vi "read.vi"(8 "error in (no error)":errorcluster, 11 "Lakeshore 336 in":refnum<class "Lakeshore 336.lvclass">) -> (0 "error out":errorcluster, 2 "Data":dbl[](array[numeric]), 3 "Lakeshore 336 out":refnum<class "Lakeshore 336.lvclass">)   [LabVIEW 2022 SP3, in "Lakeshore 336.lvclass"]
uses:
  Lakeshore 336.lvclass
  Lakeshore 336.lvclass/Lakeshore 336.ctl
  Temp Control.lvclass
  <instrlib>/Lake Shore 336/Lake Shore 336.lvlib
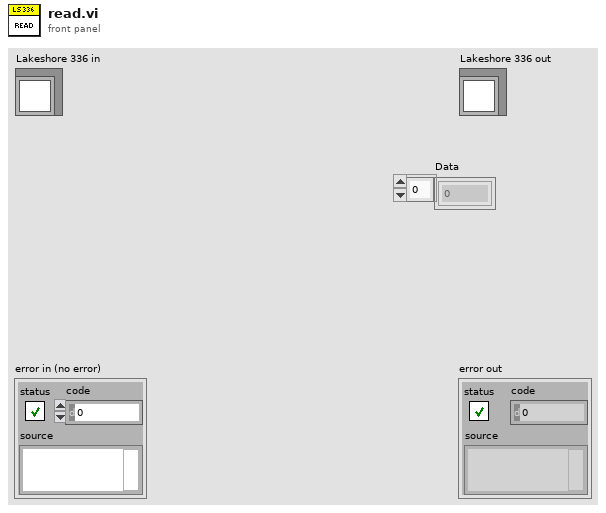
[diagram p1: front panel]
types:
  T1 = typedef "Lakeshore 336.lvclass/Lakeshore 336 Input Ch config cluster.ctl" = cluster{"Name":string}
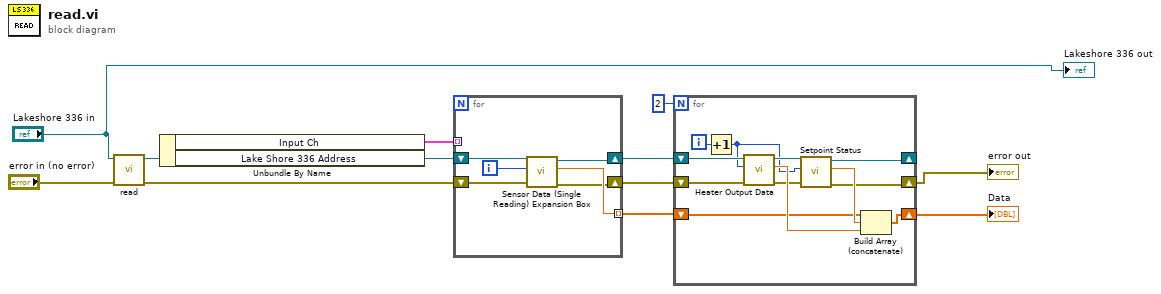
[diagram p0: block diagram]
diagram:
  n1 = call-parent "read.vi"("error in (no error)"="error in (no error)", "Temp Control in"="Lakeshore 336 in") -> ("error out"=w4:errorcluster, "Temp Control out"=w11:refnum<class "Lakeshore 336.lvclass">)  [unwired: 7 in, 1 out]
  n2 = Unbundle By Name(w11) -> ("Input Ch"=w9:T1[], "Lake Shore 336 Address"=w10:refnum<visa-resource-name>)
  n3 = for {
    tunnel: w9 -> [_] mode=indexing
    shift-right: [w16] -> w8
    shift-left: w10 -> [w18]
    tunnel: [w15] -> w6 mode=indexing
    shift-right: [w13] -> w3
    shift-left: w4 -> [w14]
    i -> [w17]
    n4 = call "Sensor Data (Single Reading) Expansion Box.vi"("error in (no error)"=w14, "Input (0:A)"=w17, "VISA resource name"=w18) -> ("error out"=w13:errorcluster, "Sensor Data"=w15:dbl, "VISA resource name out"=w16:refnum<visa-resource-name>)  [unwired: 6 in]
  }
  n5 = for {
    N: 2 -> [_]
    shift-right: [w27] -> _
    shift-left: w8 -> [w30]
    shift-right: [w23] -> w5
    shift-left: w6 -> [w24]
    shift-right: [w20] -> w2
    shift-left: w3 -> [w22]
    i -> [w29]
    n6 = Increment(x=w29) -> (x+1=w19:i32)
    n7 = call <instrlib>:"Heater Output Data.vi"("error in (no error)"=w22, "Heater Output (1:1)"=w19, "VISA resource name"=w30) -> ("error out"=w21:errorcluster, "Output Value"=w25:dbl, "VISA resource name out"=w28:refnum<visa-resource-name>)  [unwired: 6 in]
    n8 = call <instrlib>:"Setpoint Status.vi"("error in (no error)"=w21, "Output (1:1)"=w19, "VISA resource name"=w28) -> ("error out"=w20:errorcluster, "Setpoint"=w26:dbl, "VISA resource name out"=w27:refnum<visa-resource-name>)  [unwired: 6 in]
    n9 = Build Array (concatenate)(w24, w26, w25) -> (w23:dbl[])
  }
  "error out" <- w2
  "Data" <- w5
  "Lakeshore 336 out" <- "Lakeshore 336 in"
